vi "UWB Extract Position.vi"(10 "String":string, 11 "Timeout?":bool) -> (0 "Y value (mm)":i32, 3 "X value (mm)":i32)   [LabVIEW 2016]
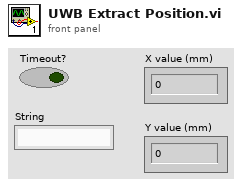
[diagram p1: front panel]
types:
  T1 = enum16{"big-endian, network order", "native, host order", "little-endian"}
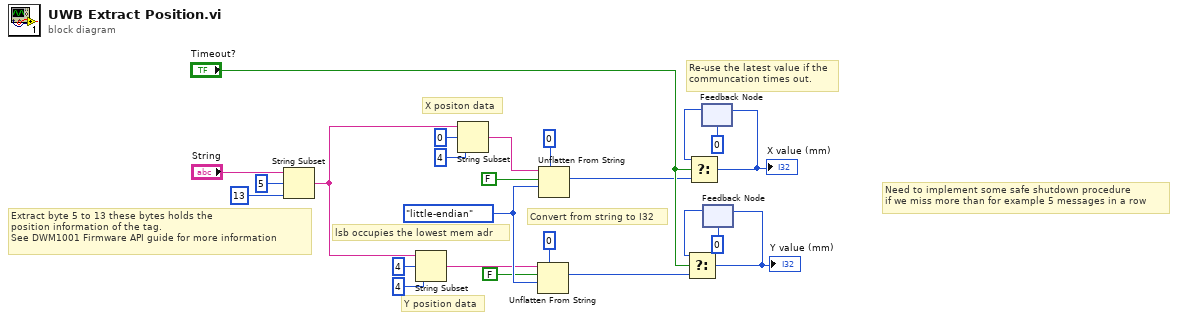
[diagram p0: block diagram]
diagram:
  w13 = T1."little-endian" ("byte order (0:big-endian, network order)")
  # "Need to implement some safe shutdown procedure\nif we miss more than for example 5 messages in a row"
  # "Re-use the latest value if the\ncommuncation times out."
  # "Convert from string to I32"
  # "lsb occupies the lowest mem adr"
  # "Y position data"
  # "X positon data"
  # "Extract byte 5 to 13 these bytes holds the \nposition information of the tag. \nSee DWM1001 Firmware API guide for more information"
  n1 = String Subset(string="String", offset (0)=5, length (rest)=13 ("length (rest)")) -> (substring=w7:string)
  n2 = String Subset(string=w7, offset (0)=4, length (rest)=4 ("length (rest)")) -> (substring=w12:string)
  n3 = String Subset(string=w7, offset (0)=0, length (rest)=4 ("length (rest)")) -> (substring=w5:string)
  n4 = Unflatten From String(type=0 ("value"), binary string=w12, data includes array or string size? (T)=FALSE, byte order (0:big-endian, network order)=w13) -> (value=w17:i32)  [unwired: 1 in, 2 out]
  n5 = Unflatten From String(type=0 ("value"), binary string=w5, data includes array or string size? (T)=FALSE, byte order (0:big-endian, network order)=w13) -> (value=w15:i32)  [unwired: 1 in, 2 out]
  n6 = feedback #1(0 ("value")) -> (w21:i32)
  n7 = Select(t=w21, s="Timeout?", f=w15) -> (s? t:f=w22:i32)
  "X value (mm)" <- w22
  n8 = feedback-in #1(w22) -> ()
  n9 = feedback #2(0 ("value")) -> (w18:i32)
  n10 = Select(t=w18, s="Timeout?", f=w17) -> (s? t:f=w19:i32)
  "Y value (mm)" <- w19
  n11 = feedback-in #2(w19) -> ()
